vi "Wave2D_Init Data_Delta.vi"(11 "Domain":T1={"t"={"initial t"=0.0, "final t"=1.0, "# of t-points"=11}, "x"={"start x"=0.0, "end x"=1.0, "# of x-points"=11}, "y"={"start y"=0.0, "end y"=1.0, "# of y-points"=11}}) -> (1 "delta y":dbl, 2 "delta x":dbl, 3 "delta t":dbl)   [LabVIEW 2017, in "NI_PDE.lvlib"]
uses:
  <vilib>/gmath/NI_PDE.lvlib
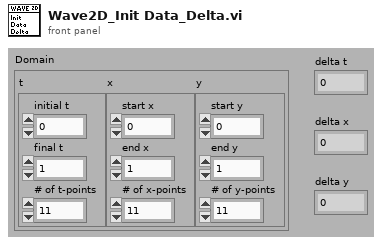
[diagram p1: front panel]
types:
  T1 = cluster{"t":cluster{"initial t":dbl, "final t":dbl, "# of t-points":i32}, "x":cluster{"start x":dbl, "end x":dbl, "# of x-points":i32}, "y":cluster{"start y":dbl, "end y":dbl, "# of y-points":i32}}
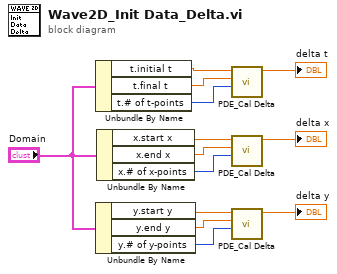
[diagram p0: block diagram]
diagram:
  n1 = Unbundle By Name("Domain") -> ("t.initial t"=w13:dbl, "t.final t"=w12:dbl, "t.# of t-points"=w11:i32)
  n2 = Unbundle By Name("Domain") -> ("y.start y"=w5:dbl, "y.end y"=w4:dbl, "y.# of y-points"=w3:i32)
  n3 = Unbundle By Name("Domain") -> ("x.start x"=w8:dbl, "x.end x"=w9:dbl, "x.# of x-points"=w10:i32)
  n4 = call <vilib>:"PDE_Cal Delta.vi"("# of points"=w11, "end"=w12, "start"=w13) -> ("delta"=→"delta t":dbl)  [unwired: 8 out]
  n5 = call <vilib>:"PDE_Cal Delta.vi"("# of points"=w10, "end"=w9, "start"=w8) -> ("delta"=→"delta x":dbl)  [unwired: 8 out]
  n6 = call <vilib>:"PDE_Cal Delta.vi"("# of points"=w3, "end"=w4, "start"=w5) -> ("delta"=→"delta y":dbl)  [unwired: 8 out]
